vi "Split_Table.vi"(0 "Table (2x2) in":u16[][](array[numeric]), 11 "error in":errorcluster caption="entrée d'erreur") -> (4 "0,0":u16, 6 "0,1":u16, 8 "1,0":u16, 10 "1,1":u16, 15 "error out":errorcluster caption="sortie d'erreur")   [LabVIEW 2023]
doc: "This vi simply separate a 2x2 table into 4 outputs"
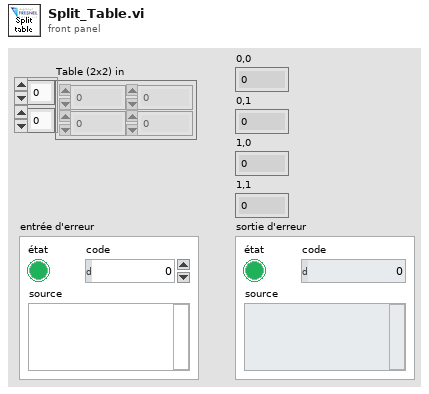
[diagram p1: front panel]
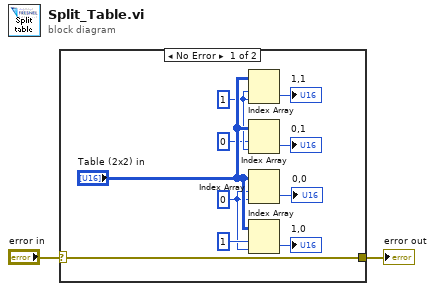
[diagram p0: block diagram]
diagram:
  n1 = case shown="No Error" "error in" {
    selector: "error in" -> [w12 w13]
    tunnel: [w12 w13] -> w1
    frame No Error {
      w6 = 1 ("disabled index (row)")
      w3 = 0 ("index (row)")
      n2 = Index Array(array="Table (2x2) in", index (row)=w6, index (col)=w6) -> (element=→"1,1":u16)
      n3 = Index Array(array="Table (2x2) in", index (row)=0, index (col)=w6) -> (element=→"0,1":u16)
      n4 = Index Array(array="Table (2x2) in", index (row)=w3, index (col)=w3) -> (element=→"0,0":u16)
      n5 = Index Array(array="Table (2x2) in", index (row)=1 ("disabled index (row)"), index (col)=w3) -> (element=→"1,0":u16)
    }
    frame Error {
    }
  }
  "error out" <- w1
